vi "WPI_Power Get PDP Faults.vi"(0 "Power Distribution Panel (0)":u8, 7 "Clear Sticky Faults":bool, 11 "error in":errorcluster) -> (4 "Current Faults":bool[](array[boolean]), 6 "Battery Voltage Fault":bool, 8 "Temperature Fault":bool, 10 "Hardware Fault":bool, 15 "error out":errorcluster)   [LabVIEW 2017]
doc: "Returns current, voltage, temp, and hardware faults on the Power Distribution Panel (PDP)."
uses:
  <vilib>/Rock Robotics/WPI/CAN/PDP/WPI_CAN_PDPGlobalOps.ctl
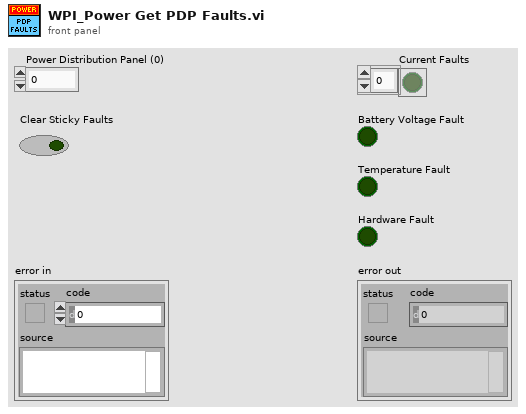
[diagram p1: front panel]
types:
  T1 = typedef "WPI_CAN_PDPGlobalOps.ctl" = enum16{"Write After Receive 0-5", "Write After Receive 6-11", "Write After Receive 12-15", "Write After Receive Energy", "Get All", "Get Commands", "Write Clear Sticky Faults Command", "Write Reset Energy Command", "Write Tare Currents Command", "Write Error", "Write After Receive Faults"}
  T2 = typedef "WPI_CAN_PDPGetAll.ctl" = cluster{"Channel Currents":dbl[], "Battery Voltage":dbl, "Temperature (degrees C)":dbl, "Internal Battery R (Ohms)":dbl, "Energy (J)":dbl, "Power (W)":dbl, "Total Current (A)":dbl, "CAN Error":errorcluster, "Current Faults":bool[], "Battery Voltage Fault":bool, "Temperature Fault":bool, "Hardware Fault":bool}
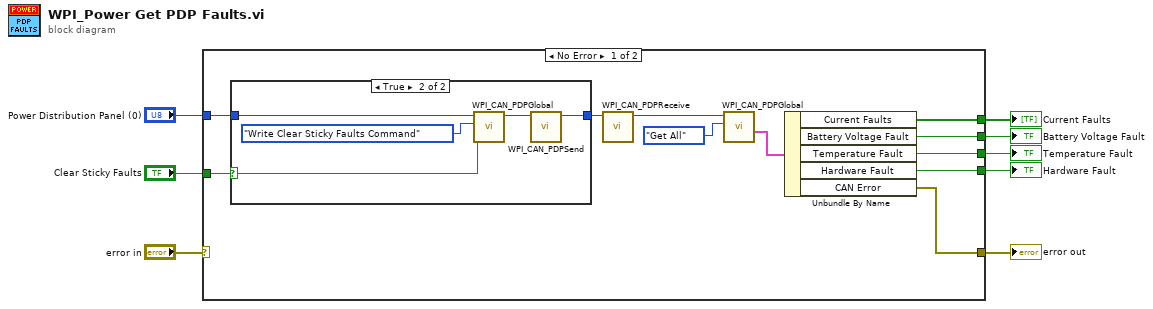
[diagram p0: block diagram]
diagram:
  n1 = case shown="No Error" "error in" {
    selector: "error in" -> [_ w26]
    tunnel: [w12 w26] -> w7
    tunnel: "Power Distribution Panel (0)" -> [w17 _]
    tunnel: [w14 _] -> w3
    tunnel: "Clear Sticky Faults" -> [w15 _]
    tunnel: [w13 _] -> w4
    tunnel: [w10 _] -> w2
    tunnel: [w9 _] -> w1
    frame No Error {
      n2 = case shown="True" w15 {
        selector: w15 -> [_ w25]
        tunnel: w17 -> [w20 w24]
        tunnel: [w20 w22] -> w16
        frame False {
        }
        frame True {
          n3 = call <vilib>:"WPI_CAN_PDPGlobal.vi"("Command"=w25, "Operation"=WPI_CAN_PDPGlobalOps."Write Clear Sticky Faults Command", "Power Distribution Panel (0)"=w24) -> ("Power Distribution Panel Out"=w23:u8)  [unwired: 6 in, 2 out]
          n4 = call <vilib>:"WPI_CAN_PDPSend.vi"("Power Distribution Panel (0)"=w23) -> ("Power Distribution Panel Out"=w22:u8)  [unwired: 10 in]
        }
      }
      n5 = call <vilib>:"WPI_CAN_PDPReceive.vi"("Power Distribution Panel (0)"=w16) -> ("Power Distribution Panel Out"=w18:u8)  [unwired: 10 in]
      n6 = call <vilib>:"WPI_CAN_PDPGlobal.vi"("Operation"=WPI_CAN_PDPGlobalOps."Get All", "Power Distribution Panel (0)"=w18) -> ("Get All"=w19:T2)  [unwired: 7 in, 2 out]
      n7 = Unbundle By Name(w19) -> ("Current Faults"=w13:bool[], "Battery Voltage Fault"=w14:bool, "Temperature Fault"=w10:bool, "Hardware Fault"=w9:bool, "CAN Error"=w12:errorcluster)
    }
    frame Error {
    }
  }
  "error out" <- w7
  "Current Faults" <- w4
  "Battery Voltage Fault" <- w3
  "Temperature Fault" <- w2
  "Hardware Fault" <- w1
